vi "Cartridge Mngr.vi"(5 "Main References":T4, 7 "Mngr Action":T5, 8 "error in (no error)":errorcluster, 10 "Cartrdige #":i32) -> (0 "error out":errorcluster, 2 "Current State":T3=enum."Lock", 3 "Cartridges":T1)   [LabVIEW 2018]
uses:
  Cartridge Mngr.ctl
  Main Refs.ctl
  Hardware/Tecan/Pump Config.ctl
  Vacuum Specs.ctl
  Timing Specs.ctl
  Cartridges.ctl
  Cartridge Status.ctl
  Commands.ctl
  Lib/Time/Wells.ctl
  Lib/Time/Bottles.ctl
  Process State.ctl
  Vacuum Test.ctl
  Cartridge state.ctl
  Hardware/DAQ Mngr.ctl
  Hardware/NFC Mngr.ctl
panel:
  # "Tecan Pump"
  # "Vacuum"
  # "General"
  # "Timing"
  # "Protocol"
  # "Zaber"
  # "NFC Reader 1"
  # "NFC  Reader 2"
  # "NFC Reader 3"
  # "NFC Reader 4"
  # "System"
  # "Cartridge Utitlies"
  # "Wells"
  # "times"
  # "from"
  # "State Machine"
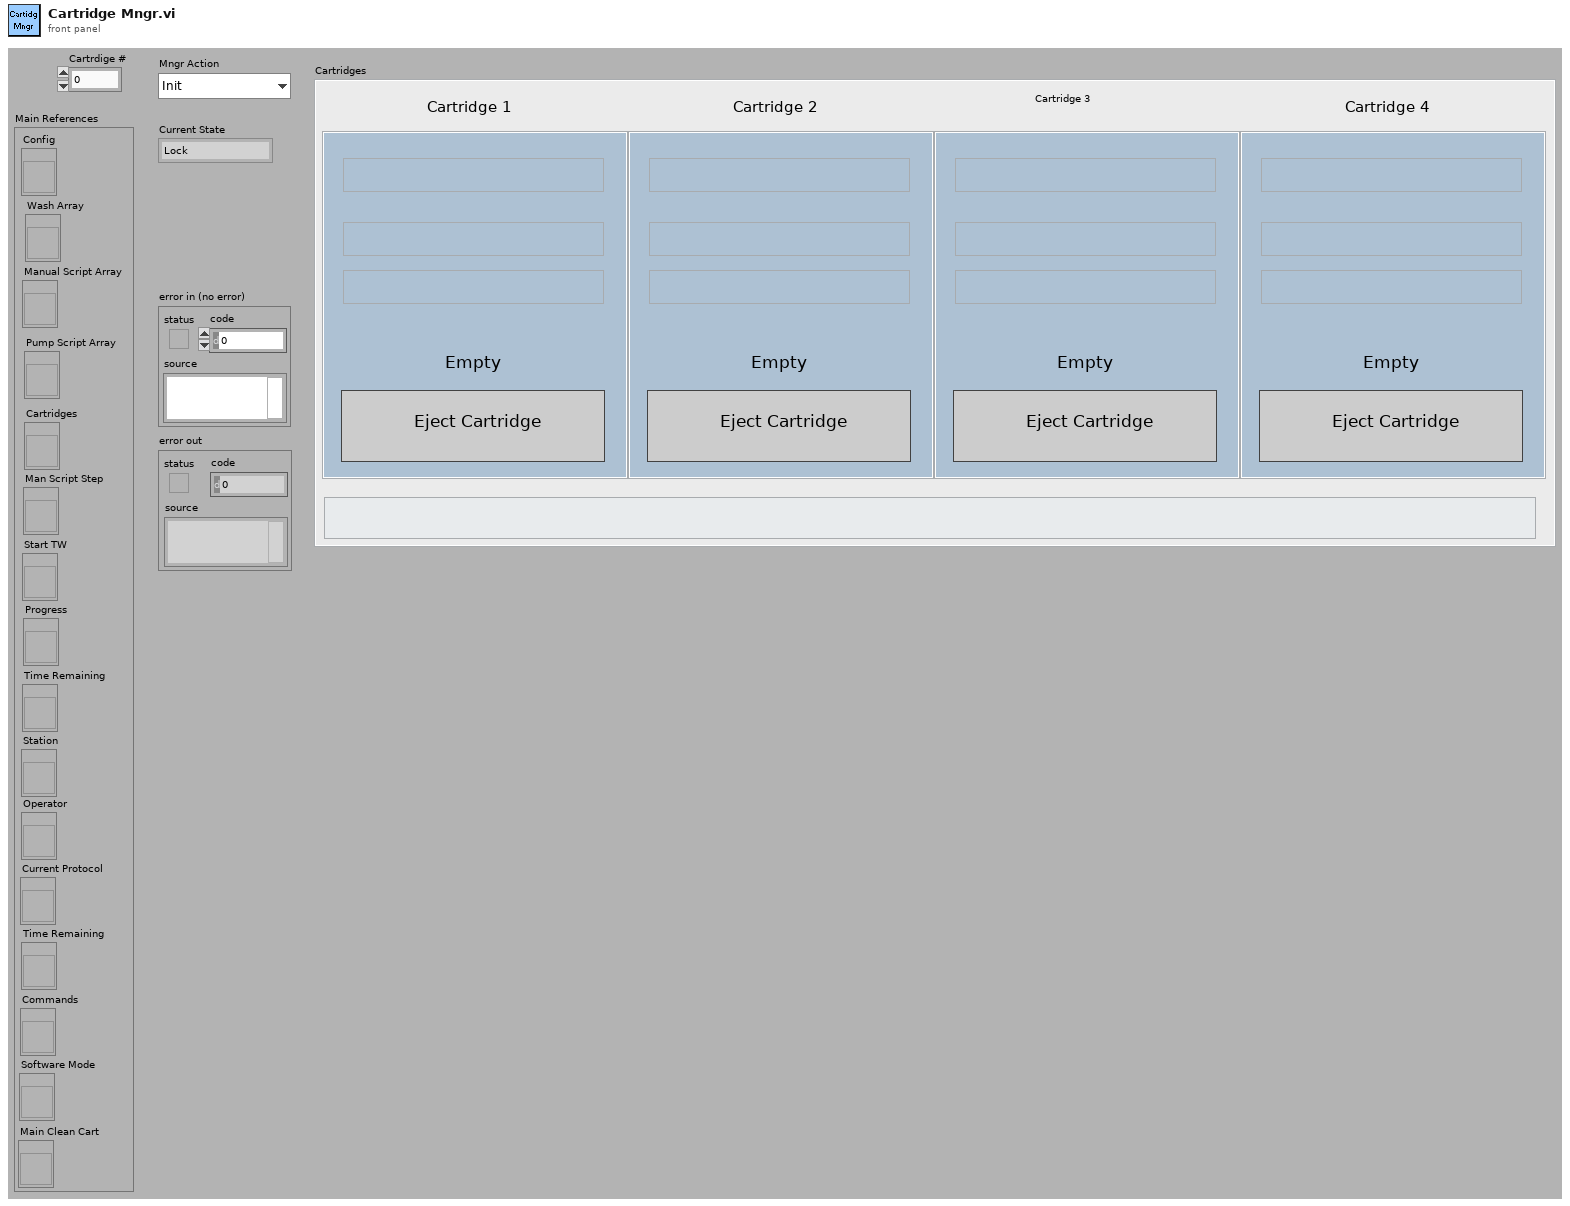
[diagram p1: front panel]
types:
  T1 = typedef "Cartridges.ctl" = cluster{"Cartridge 1":T2, "Cartridge 2":T2, "Cartridge 3":T2, "Cartridge 4":T2, "Current Status":string}
  T2 = typedef "Cartridge Status.ctl" = cluster{"Serial Number":string, "Reagent":string, "Cart Status":string, "Inserted":bool, "Eject":bool}
  T3 = typedef "Cartridge state.ctl" = enum16{"Init", "Detect", "Lock", "Read SN", "Unlock", "Error"}
  T4 = typedef "Main Refs.ctl" = cluster{"Config":refnum<vi>, "Wash Array":refnum<vi>, "Manual Script Array":refnum<vi>, "Pump Script Array":refnum<vi>, "Cartridges":refnum<vi>, "Man Script Step":refnum<vi>, "Start TW":refnum<vi>, "Progress":refnum<vi>, "Time Remaining":refnum<vi>, "Station":refnum<vi>, "Operator":refnum<vi>, "Current Protocol":refnum<vi>, "Time Remaining":refnum<vi>, "Commands":refnum<vi>, "Software Mode":refnum<vi>, "Main Clean Cart":refnum<vi>}
  T5 = typedef "Cartridge Mngr.ctl" = enum16{"Init", "Update", "Detect", "Lock", "Read SN", "Unlock", "Error"}
  T6 = typedef "DAQ Mngr.ctl" = enum16{"Init", "Read Vacuum", "Analyze Vacuum", "Read Cartridges", "Lock Cartridge", "Unlock Cartridge", "Read PS", "Pinch Valve Engage", "Pinch Valve Disengage", "Close"}
  T7 = typedef "NFC Mngr.ctl" = enum16{"Connect", "Read SN", "Close"}
  T8 = enum8{"Enabled", "Disabled", "Disabled and Grayed Out"}
  T9 = typedef "Pump Config.ctl" = cluster{"Syringe size":u32, "Syringe address":u32, "# of ports":u32, "Init String":string, "Full Stroke (cnts)":i32, "Model":enum16{"XC", "Centris"}, "TW Position":dbl, "Load Position":dbl, "Bottom Position":dbl, "Station ID":string, "Vacuum Specs":T10, "Default Protocol":path, "Dry Time(s)":dbl, "Python Version":string, "NFC SN Array":string[], "Timing":T11}
  T10 = typedef "Vacuum Specs.ctl" = cluster{"vacuum max":dbl, "vacuum min":dbl, "liq2air rate delta":dbl, "liq2air time":dbl, "Conf. R":dbl, "LeakRateMax":dbl}
  T11 = typedef "Timing Specs.ctl" = cluster{"Checking vac and leak":dbl, "Priming input lines":dbl, "Rinsing syringe":dbl, "Filling well X w/ X":dbl, "Drain well X":dbl, "Clearing wells and lines":dbl, "Draining wells":dbl, "Rinsing all wells":dbl, "Testing for leaks/clogs":dbl, "Rinsing wells":dbl}
  T12 = cluster{"negative limit switch":bool, "positive limit switch":bool, "home switch":bool, "position marker":bool, "device enable":bool, "quick stop":bool, "general purpose J":bool, "general purpose I":bool, "general purpose H":bool, "general purpose G":bool, "general purpose F":bool, "general purpose E":bool, "general purpose D":bool, "general purpose C":bool, "general purpose B":bool, "general purpose A":bool}
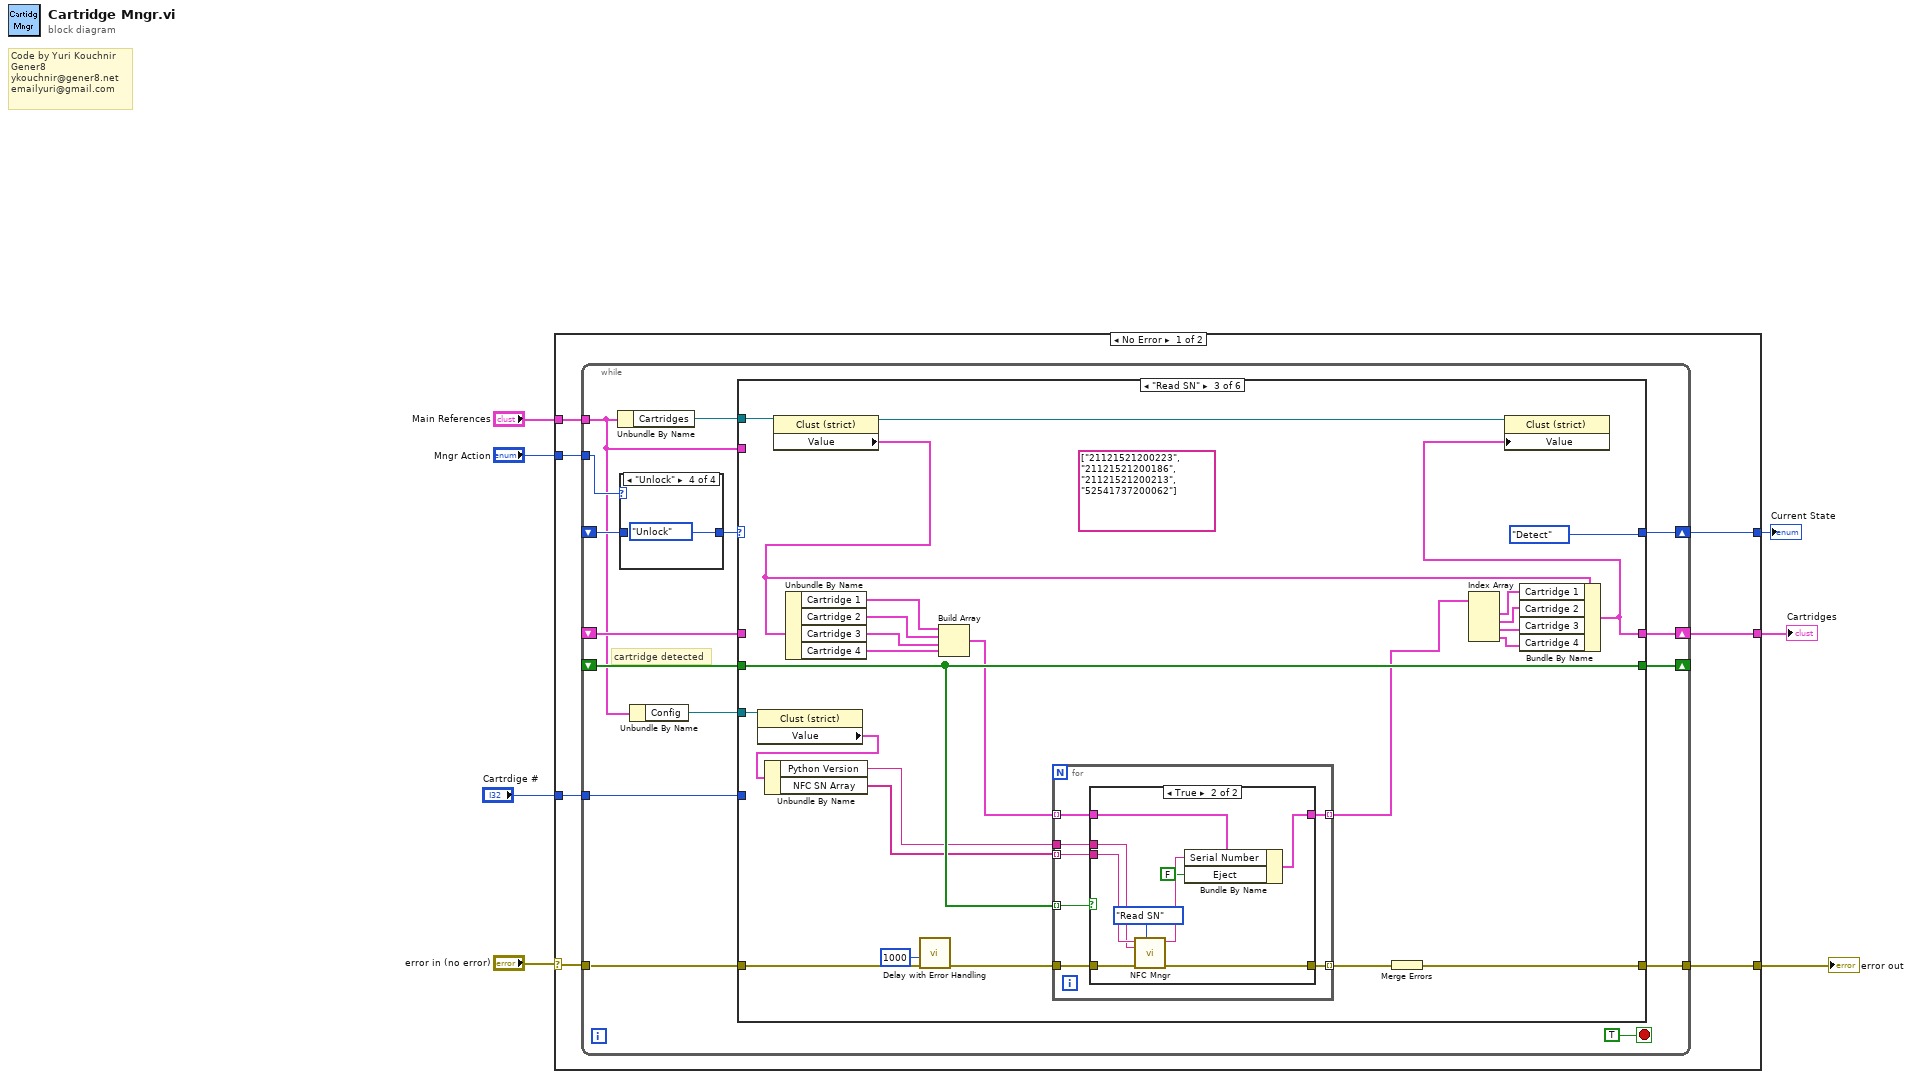
[diagram p0: block diagram]
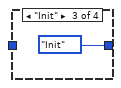
[diagram p4: hidden frame]
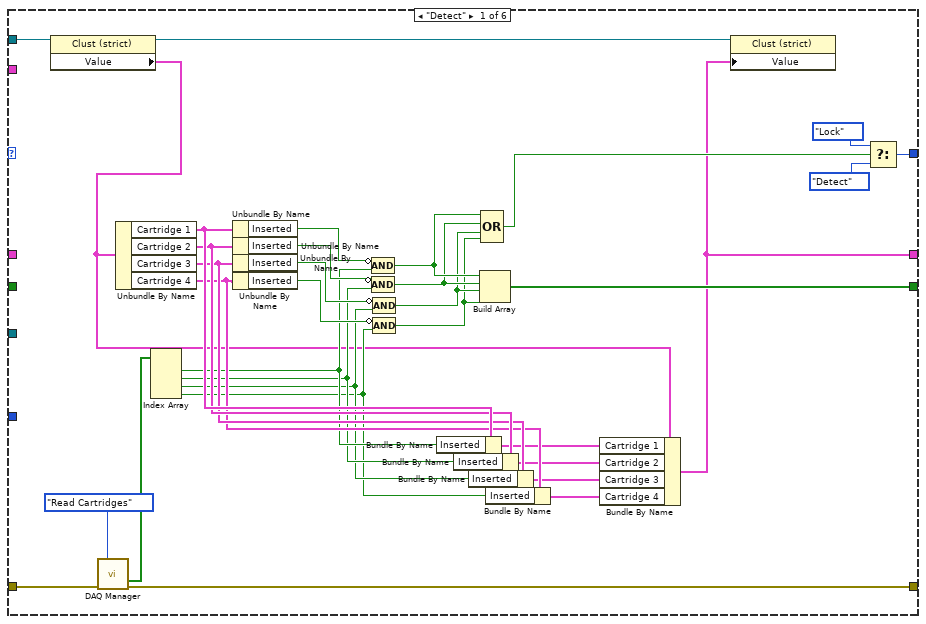
[diagram p5: hidden frame]
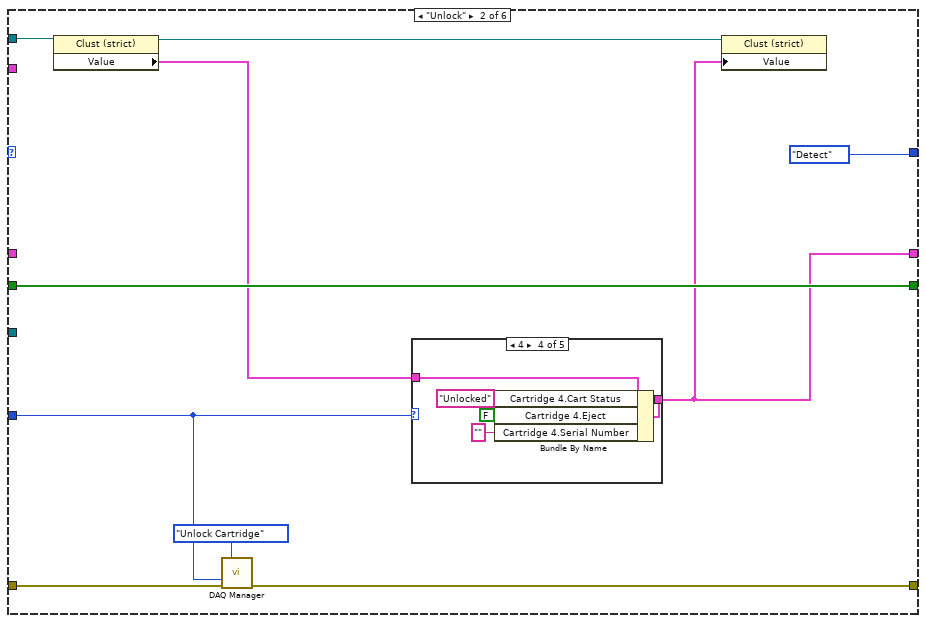
[diagram p6: hidden frame]
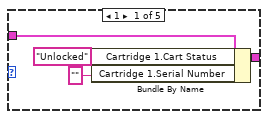
[diagram p7: hidden frame]
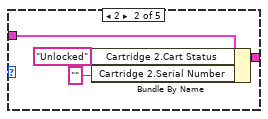
[diagram p8: hidden frame]
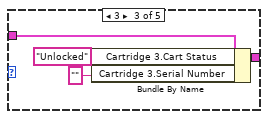
[diagram p9: hidden frame]
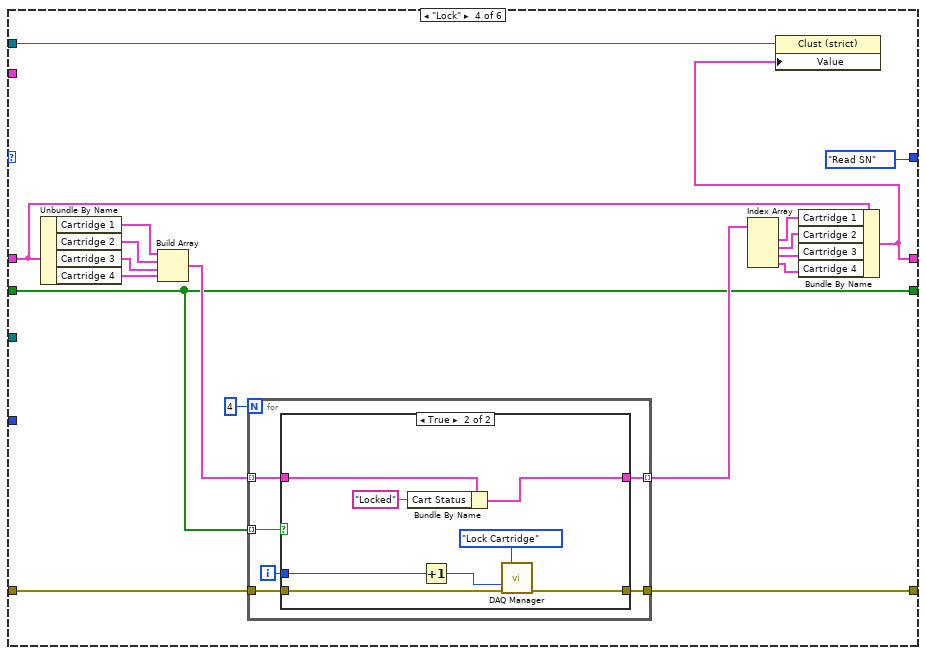
[diagram p12: hidden frame]
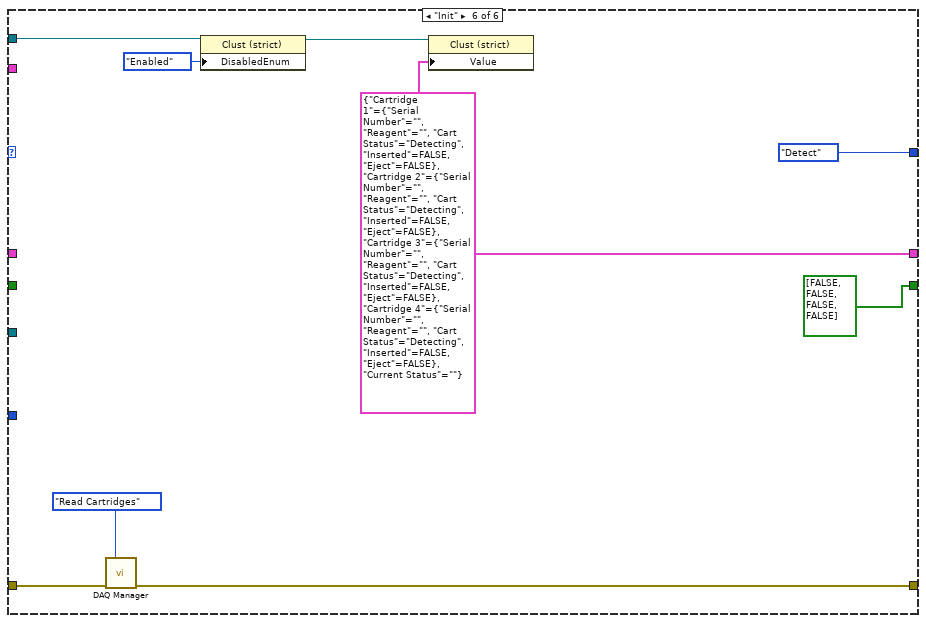
[diagram p15: hidden frame]
diagram:
  # "Code by Yuri Kouchnir\nGener8\nykouchnir@gener8.net\nemailyuri@gmail.com"
  n1 = case shown="No Error" "error in (no error)" {
    selector: "error in (no error)" -> [w14 w185]
    tunnel: [w13 w185] -> w6
    tunnel: "Mngr Action" -> [w12 _]
    tunnel: "Main References" -> [w11 _]
    tunnel: "Cartrdige #" -> [w10 _]
    tunnel: [w9 _] -> w2
    tunnel: [w8 _] -> w1
    frame No Error {
      n2 = while {
        tunnel: w14 -> [w28]
        tunnel: [w27] -> w13
        tunnel: w12 -> [w23]
        shift-right: [w26] -> w9
        shift-left: _ -> [w25]
        tunnel: w11 -> [w16]
        shift-right: [w21] -> w8
        shift-left: _ -> [w20]
        shift-right: [w19] -> _
        shift-left: _ -> [w18]
        tunnel: w10 -> [w17]
        stop <- TRUE stop-if-true
        # "cartridge detected"
        n3 = Unbundle By Name(w16) -> ("Cartridges"=w22:refnum<vi>)
        n4 = case shown="\"Unlock\"" w23 {
          tunnel: w25 -> [w30 w31 _ _]
          tunnel: [w30 w31 Cartridge_state."Init" ("State") Cartridge_state."Unlock" ("State")] -> w24
          frame Default {
          }
          frame "Update" {
          }
          frame "Init" {
          }
          frame "Unlock" {
          }
        }
        n5 = Unbundle By Name(w16) -> ("Config"=w15:refnum<vi>)
        n6 = case shown="\"Read SN\"" w24 {
          selector: w24 -> [_ _ _ _ w175 _]
          tunnel: w28 -> [w66 w76 w119 w155 w172 w180]
          tunnel: [w65 w75 w95 w154 w172 w179] -> w27
          tunnel: [w58 Cartridge_state."Detect" ("State") Cartridge_state."Detect" ("State") Cartridge_state."Read SN" ("State") w175 Cartridge_state."Detect" ("State")] -> w26
          tunnel: w22 -> [w36 w70 w104 w148 _ w183]
          tunnel: [w37 w67 w109 w140 w174 w182] -> w21
          tunnel: w20 -> [_ _ _ w146 w174 _]
          tunnel: [w57 w74 w107 w139 w173 bool[] [FALSE, FALSE, FALSE, FALSE]] -> w19
          tunnel: w18 -> [_ w74 w107 w139 w173 _]
          tunnel: w17 -> [_ w71 _ _ _ _]
          tunnel: w16 -> [_ _ _ _ _ _]
          tunnel: w15 -> [_ _ w100 _ _ _]
          frame "Detect" {
            n7 = property class="Clust (strict)"(reference=w36) -> (reference out=w34:refnum<vi>, "Value"=w35:T1)  [unwired: 1 in, 1 out]
            n8 = call "DAQ Manager.vi"("DAQ Mngr Action"=DAQ_Mngr."Read Cartridges", "error in (no error)"=w66) -> ("Cart Sense"=w56:bool[], "error out"=w65:errorcluster)  [unwired: 7 in, 5 out]
            n9 = Unbundle By Name(w35) -> ("Cartridge 1"=w49:T2, "Cartridge 2"=w48:T2, "Cartridge 3"=w47:T2, "Cartridge 4"=w46:T2)
            n10 = Index Array(array=w56) -> (element #1=w41:bool, element #2=w40:bool, element #3=w39:bool, element #4=w38:bool)  [unwired: 4 in]
            n11 = Unbundle By Name(w49) -> ("Inserted"=w53:bool)
            n12 = Unbundle By Name(w48) -> ("Inserted"=w52:bool)
            n13 = Unbundle By Name(w47) -> ("Inserted"=w51:bool)
            n14 = Unbundle By Name(w46) -> ("Inserted"=w50:bool)
            n15 = Compound Arithmetic op=AND(invert w53, w41) -> (w63:bool)
            n16 = Compound Arithmetic op=AND(invert w52, w40) -> (w62:bool)
            n17 = Compound Arithmetic op=AND(invert w51, w39) -> (w61:bool)
            n18 = Compound Arithmetic op=AND(invert w50, w38) -> (w60:bool)
            n19 = Bundle By Name(cluster=w49, "Inserted"=w41) -> (w45:T2)
            n20 = Bundle By Name(cluster=w48, "Inserted"=w40) -> (w44:T2)
            n21 = Bundle By Name(cluster=w47, "Inserted"=w39) -> (w43:T2)
            n22 = Build Array(w63, w62, w61, w60) -> (w57:bool[])
            n23 = Compound Arithmetic op=OR(w63, w62, w61, w60) -> (w59:bool)
            n24 = Bundle By Name(cluster=w46, "Inserted"=w38) -> (w42:T2)
            n25 = Bundle By Name(cluster=w35, "Cartridge 1"=w45, "Cartridge 2"=w44, "Cartridge 3"=w43, "Cartridge 4"=w42) -> (w37:T1)
            n26 = property class="Clust (strict)"(reference=w34, "Value"=w37) -> ()  [unwired: 1 in, 2 out]
            n27 = Select(t=Cartridge_state."Lock" ("State"), s=w59, f=Cartridge_state."Detect" ("State")) -> (s? t:f=w58:T3)
          }
          frame "Unlock" {
            n28 = property class="Clust (strict)"(reference=w70) -> (reference out=w68:refnum<vi>, "Value"=w69:T1)  [unwired: 1 in, 1 out]
            n29 = call "DAQ Manager.vi"("DAQ Mngr Action"=DAQ_Mngr."Unlock Cartridge", "Value"=w71, "error in (no error)"=w76) -> ("error out"=w75:errorcluster)  [unwired: 6 in, 6 out]
            n30 = case shown="4" w71 {
              tunnel: w69 -> [w80 w84 w88 w93 w94]
              tunnel: [w79 w83 w87 w92 w94] -> w67
              frame 1 {
                n31 = Bundle By Name(cluster=w80, "Cartridge 1.Cart Status"="Unlocked" ("Cart Status"), "Cartridge 1.Serial Number"="") -> (w79:T1)
              }
              frame 2 {
                n32 = Bundle By Name(cluster=w84, "Cartridge 2.Cart Status"="Unlocked" ("Cart Status"), "Cartridge 2.Serial Number"="") -> (w83:T1)
              }
              frame 3 {
                n33 = Bundle By Name(cluster=w88, "Cartridge 3.Cart Status"="Unlocked" ("Cart Status"), "Cartridge 3.Serial Number"="") -> (w87:T1)
              }
              frame 4 {
                n34 = Bundle By Name(cluster=w93, "Cartridge 4.Cart Status"="Unlocked" ("Cart Status"), "Cartridge 4.Eject"=FALSE, "Cartridge 4.Serial Number"="") -> (w92:T1)
              }
              frame Default {
              }
            }
            n35 = property class="Clust (strict)"(reference=w68, "Value"=w67) -> ()  [unwired: 1 in, 2 out]
          }
          frame "Read SN" {
            (unwired) string[] ["21121521200223", "21121521200186", "21121521200213", "52541737200062"]
            n36 = property class="Clust (strict)"(reference=w100) -> ("Value"=w99:T9)  [unwired: 1 in, 2 out]
            n37 = Unbundle By Name(w99) -> ("Python Version"=w97:string, "NFC SN Array"=w98:string[])
            n38 = property class="Clust (strict)"(reference=w104) -> (reference out=w102:refnum<vi>, "Value"=w103:T1)  [unwired: 1 in, 1 out]
            n39 = Unbundle By Name(w103) -> ("Cartridge 1"=w117:T2, "Cartridge 2"=w116:T2, "Cartridge 3"=w115:T2, "Cartridge 4"=w114:T2)
            n40 = call "Delay with Error Handling.vi"("error in (no error)"=w119, "Delay (ms)"=u32 1000) -> ("error out"=w96:errorcluster)  [unwired: 9 in]
            n41 = Build Array(w117, w116, w115, w114) -> (w105:T2[])
            n42 = for {
              tunnel: [w125] -> w106 mode=indexing
              tunnel: w107 -> [w124] mode=indexing
              tunnel: w105 -> [w123] mode=indexing
              tunnel: w98 -> [w122] mode=indexing
              tunnel: w97 -> [w121]
              tunnel: w96 -> [w120]
              tunnel: [w126] -> w118 mode=indexing
              n43 = case shown="True" w124 {
                tunnel: w120 -> [w128 w135]
                tunnel: [w128 w132] -> w126
                tunnel: [w127 w136] -> w125
                tunnel: w123 -> [w127 w137]
                tunnel: w122 -> [_ w134]
                tunnel: w121 -> [_ w129]
                frame False {
                }
                frame True {
                  n44 = call "NFC Mngr.vi"("Mngr Action"=NFC_Mngr."Read SN", "error in (no error)"=w135, "Python Version"=w129, "Reader SN"=w134) -> ("error out"=w132:errorcluster, "Cartridge SN"=w133:string)  [unwired: 5 in, 1 out]
                  n45 = Bundle By Name(cluster=w137, "Serial Number"=w133, "Eject"=FALSE) -> (w136:T2)
                }
              }
            }
            n46 = Merge Errors(w118) -> (w95:errorcluster)
            n47 = Index Array(array=w106) -> (element #1=w113:T2, element #2=w112:T2, element #3=w111:T2, element #4=w110:T2)  [unwired: 4 in]
            n48 = Bundle By Name(cluster=w103, "Cartridge 1"=w113, "Cartridge 2"=w112, "Cartridge 3"=w111, "Cartridge 4"=w110) -> (w109:T1)
            n49 = property class="Clust (strict)"(reference=w102, "Value"=w109) -> ()  [unwired: 1 in, 2 out]
          }
          frame "Lock" {
            n50 = Unbundle By Name(w146) -> ("Cartridge 1"=w152:T2, "Cartridge 2"=w151:T2, "Cartridge 3"=w150:T2, "Cartridge 4"=w149:T2)
            n51 = Build Array(w152, w151, w150, w149) -> (w147:T2[])
            n52 = for {
              N: 4 -> [_]
              tunnel: w155 -> [w161]
              tunnel: [w160] -> w154
              tunnel: w139 -> [w159] mode=indexing
              tunnel: [w158] -> w145 mode=indexing
              tunnel: w147 -> [w157] mode=indexing
              i -> [w156]
              n53 = case shown="True" w159 {
                tunnel: w161 -> [w163 w171]
                tunnel: [w163 w170] -> w160
                tunnel: [w162 w164] -> w158
                tunnel: w157 -> [w162 w166]
                tunnel: w156 -> [_ w169]
                frame False {
                }
                frame True {
                  n54 = Bundle By Name(cluster=w166, "Cart Status"="Locked") -> (w164:T2)
                  n55 = Increment(x=w169) -> (x+1=w167:i32)
                  n56 = call "DAQ Manager.vi"("DAQ Mngr Action"=DAQ_Mngr."Lock Cartridge", "Value"=w167, "error in (no error)"=w171) -> ("error out"=w170:errorcluster)  [unwired: 6 in, 6 out]
                }
              }
            }
            n57 = Index Array(array=w145) -> (element #1=w144:T2, element #2=w143:T2, element #3=w142:T2, element #4=w141:T2)  [unwired: 4 in]
            n58 = Bundle By Name(cluster=w146, "Cartridge 1"=w144, "Cartridge 2"=w143, "Cartridge 3"=w142, "Cartridge 4"=w141) -> (w140:T1)
            n59 = property class="Clust (strict)"(reference=w148, "Value"=w140) -> ()  [unwired: 1 in, 2 out]
          }
          frame "Error" {
          }
          frame "Init" {
            w182 = T1 {"Cartridge 1"={"Serial Number"="", "Reagent"="", "Cart Status"="Detecting", "Inserted"=FALSE, "Eject"=FALSE}, "Cartridge 2"={"Serial Number"="", "Reagent"="", "Cart Status"="Detecting", "Inserted"=FALSE, "Eject"=FALSE}, "Cartridge 3"={"Serial Number"="", "Reagent"="", "Cart Status"="Detecting", "Inserted"=FALSE, "Eject"=FALSE}, "Cartridge 4"={"Serial Number"="", "Reagent"="", "Cart Status"="Detecting", "Inserted"=FALSE, "Eject"=FALSE}, "Current Status"=""} ("Value")
            n60 = call "DAQ Manager.vi"("DAQ Mngr Action"=DAQ_Mngr."Read Cartridges", "error in (no error)"=w180) -> ("error out"=w179:errorcluster)  [unwired: 7 in, 6 out]
            n61 = property class="Clust (strict)"(reference=w183, "DisabledEnum"=T8."Enabled" ("Disabled")) -> (reference out=w181:refnum<vi>)  [unwired: 1 in, 1 out]
            n62 = property class="Clust (strict)"(reference=w181, "Value"=w182) -> ()  [unwired: 1 in, 2 out]
          }
        }
      }
    }
    frame Error {
      (unwired) T12 {"negative limit switch"=FALSE, "positive limit switch"=FALSE, "home switch"=FALSE, "position marker"=FALSE, "device enable"=FALSE, "quick stop"=FALSE, "general purpose J"=FALSE, "general purpose I"=FALSE, "general purpose H"=FALSE, "general purpose G"=FALSE, "general purpose F"=FALSE, "general purpose E"=FALSE, "general purpose D"=FALSE, "general purpose C"=FALSE, "general purpose B"=FALSE, "general purpose A"=FALSE} ("digital inputs")
    }
  }
  "error out" <- w6
  "Current State" <- w2
  "Cartridges" <- w1
